vi "Measure the Function on 1st Display.vi"(5 "Type for Temperature":u8(ring) items=["J Type", "K Type", "T Type"], 7 "Manual Range":dbl format="%#.9e", 8 "error in":errorcluster, 9 "Enable Auto Range":bool=TRUE, 10 "Function":u8(ring) items=["DC Voltage", "AC Voltage", "DC+AC Voltage", "DC Current", "AC Current", "DC+AC Current", "2-Wire Resistance", "Frequency", "Period", "Continuity", "Diode", "Temperature", "Capacitance"], 11 "VISA resource name":refnum<visa-resource-name>) -> (0 "error out":errorcluster, 2 "Return the Value":string, 3 "VISA resource name out":refnum<visa-resource-name>)   [LabVIEW 2011, in "DMM4.lvlib"]
uses:
  <instrlib>/DMM4/DMM4.lvlib
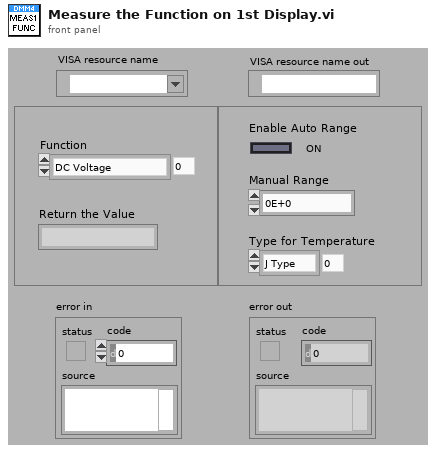
[diagram p1: front panel]
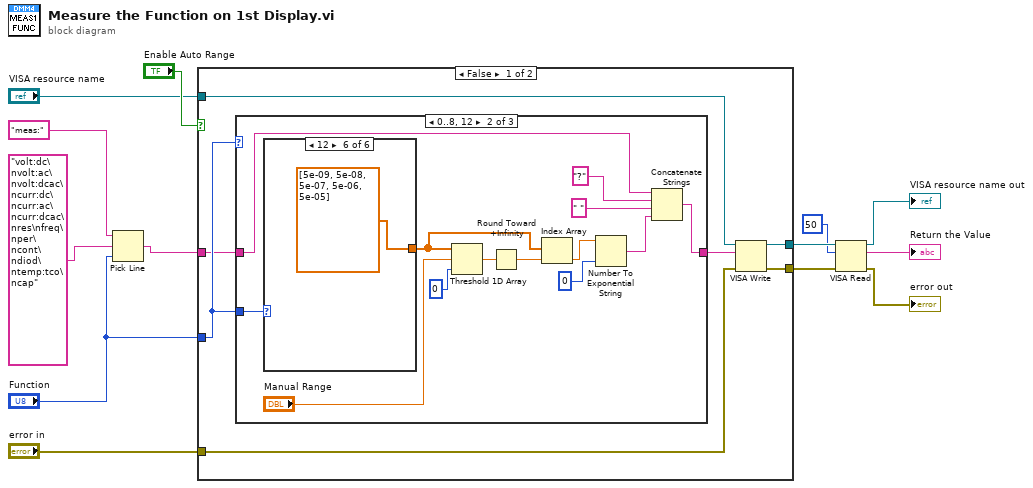
[diagram p0: block diagram]
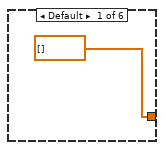
[diagram p3: hidden frame]
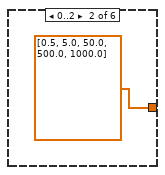
[diagram p4: hidden frame]
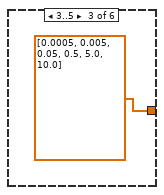
[diagram p5: hidden frame]
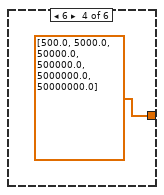
[diagram p6: hidden frame]
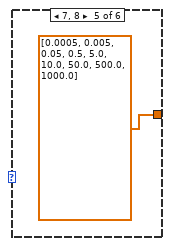
[diagram p7: hidden frame]
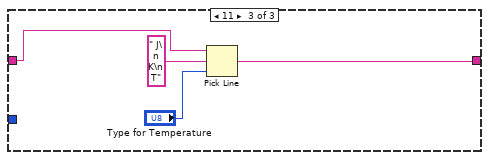
[diagram p8: hidden frame]
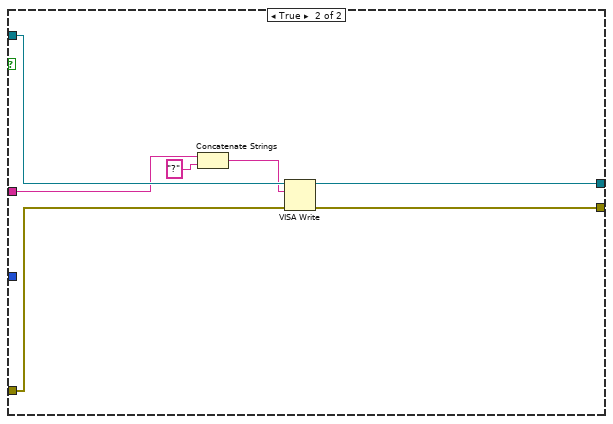
[diagram p9: hidden frame]
diagram:
  n1 = Pick Line(string ("")="meas:", multi-line string="volt:dc\nvolt:ac\nvolt:dcac\ncurr:dc\ncurr:ac\ncurr:dcac\nres\nfreq\nper\ncont\ndiod\ntemp:tco\ncap", line index="Function") -> (output string=w9:string)
  n2 = case shown="False" "Enable Auto Range" {
    tunnel: "Function" -> [w20 _]
    tunnel: w9 -> [w19 w47]
    tunnel: "VISA resource name" -> [w17 w51]
    tunnel: "error in" -> [w16 w50]
    tunnel: [w15 w49] -> w6
    tunnel: [w14 w48] -> w5
    frame False {
      n3 = case shown="0..8, 12" w20 {
        tunnel: w20 -> [_ w24 _]
        tunnel: w19 -> [w21 w23 w41]
        tunnel: [w21 w25 w42] -> w18
        frame Default {
        }
        frame 0..8, 12 {
          n4 = case shown="12" w24 {
            tunnel: [dbl[] [] dbl[] [0.5, 5.0, 50.0, 500.0, 1000.0] dbl[] [0.0005, 0.005, 0.05, 0.5, 5.0, 10.0] dbl[] [500.0, 5000.0, 50000.0, 500000.0, 5000000.0, 50000000.0] dbl[] [0.0005, 0.005, 0.05, 0.5, 5.0, 10.0, 50.0, 500.0, 1000.0] dbl[] [5e-09, 5e-08, 5e-07, 5e-06, 5e-05]] -> w30
            frame Default {
            }
            frame 0..2 {
            }
            frame 3..5 {
            }
            frame 6 {
            }
            frame 7, 8 {
            }
            frame 12 {
            }
          }
          n5 = Threshold 1D Array(1:0 ("start index (0)"), 2:"Manual Range", 3:w30) -> (0:w32:dbl)
          n6 = Round Toward +Infinity(x=w32) -> (ceil(x): smallest int >= x=w31:dbl)
          n7 = Index Array(array=w30, index=w31) -> (element=w29:dbl)
          n8 = Number To Exponential String(number=w29, precision (6)=i16 0) -> (E-format string=w26:string)  [unwired: 2 in]
          n9 = Concatenate Strings(w23, "?" ("string"), " " ("string"), w26) -> (w25:string)
        }
        frame 11 {
          n10 = Pick Line(string ("")=w41, multi-line string=" J\n K\n T", line index="Type for Temperature") -> (output string=w42:string)
        }
      }
      n11 = VISA Write(VISA resource name=w17, write buffer=w18, error in (no error)=w16) -> (VISA resource name out=w15:refnum<visa-resource-name>, error out=w14:errorcluster)  [unwired: 1 out]
    }
    frame True {
      n12 = Concatenate Strings(w47, "?" ("string")) -> (w45:string)
      n13 = VISA Write(VISA resource name=w51, write buffer=w45, error in (no error)=w50) -> (VISA resource name out=w49:refnum<visa-resource-name>, error out=w48:errorcluster)  [unwired: 1 out]
    }
  }
  n14 = VISA Read(VISA resource name=w6, byte count=u32 50, error in (no error)=w5) -> (VISA resource name out=→"VISA resource name out":refnum<visa-resource-name>, read buffer=→"Return the Value":string, error out=→"error out":errorcluster)  [unwired: 1 out]
